vi "default scan size.vi"(0 "data in":T1, 11 "error in":errorcluster) -> (4 "data out":T1, 15 "error out":errorcluster)   [LabVIEW 2013, in "Manipulate IPF.lvlib"]
uses:
  Manipulate IPF.lvlib
  3013/code/Modules/GUI/GUI_5/subPanels/edit/type_def/data.ctl
  3013/code/Modules/Configuration/type_def/Scan Params.ctl
  3013/code/Modules/Configuration/type_def/Profile Resolution.ctl
  3013/code/Modules/Preprocess Data/type_def/direction.ctl
  3013/code/Modules/Inspection/Data/Panel_class/type_def/Config File data.ctl
  3013/code/Modules/Inspection/type_def/Pos and Rot.ctl
  3013/code/Modules/Inspection/Data/PCB_class/type_def/PCB Params.ctl
  3013/code/Modules/Inspection/Data/Panel_class/type_def/BarCode Params.ctl
  3013/code/Modules/Barcode Reader/type_def/id.ctl
  3013/code/Modules/Inspection/Data/Panel_class/type_def/inspection data.ctl
  3013/code/Modules/Inspection/type_def/Range Limits.ctl
  3013/code/Modules/Configuration/Config.lvlib
  3013/code/Modules/Inspection/Inspection.lvlib
  3013/code/Modules/Inspection/Data/PCB_class/PCB.lvclass
  3013/code/Modules/Barcode Reader/Barcode Reader.lvlib
  3013/code/Modules/Inspection/Data/Panel_class/Panel.lvclass
  3013/code/Modules/Preprocess Data/PreProcess.lvlib
  3013/code/Modules/GUI/GUI_5/subPanels/edit/edit.lvlib
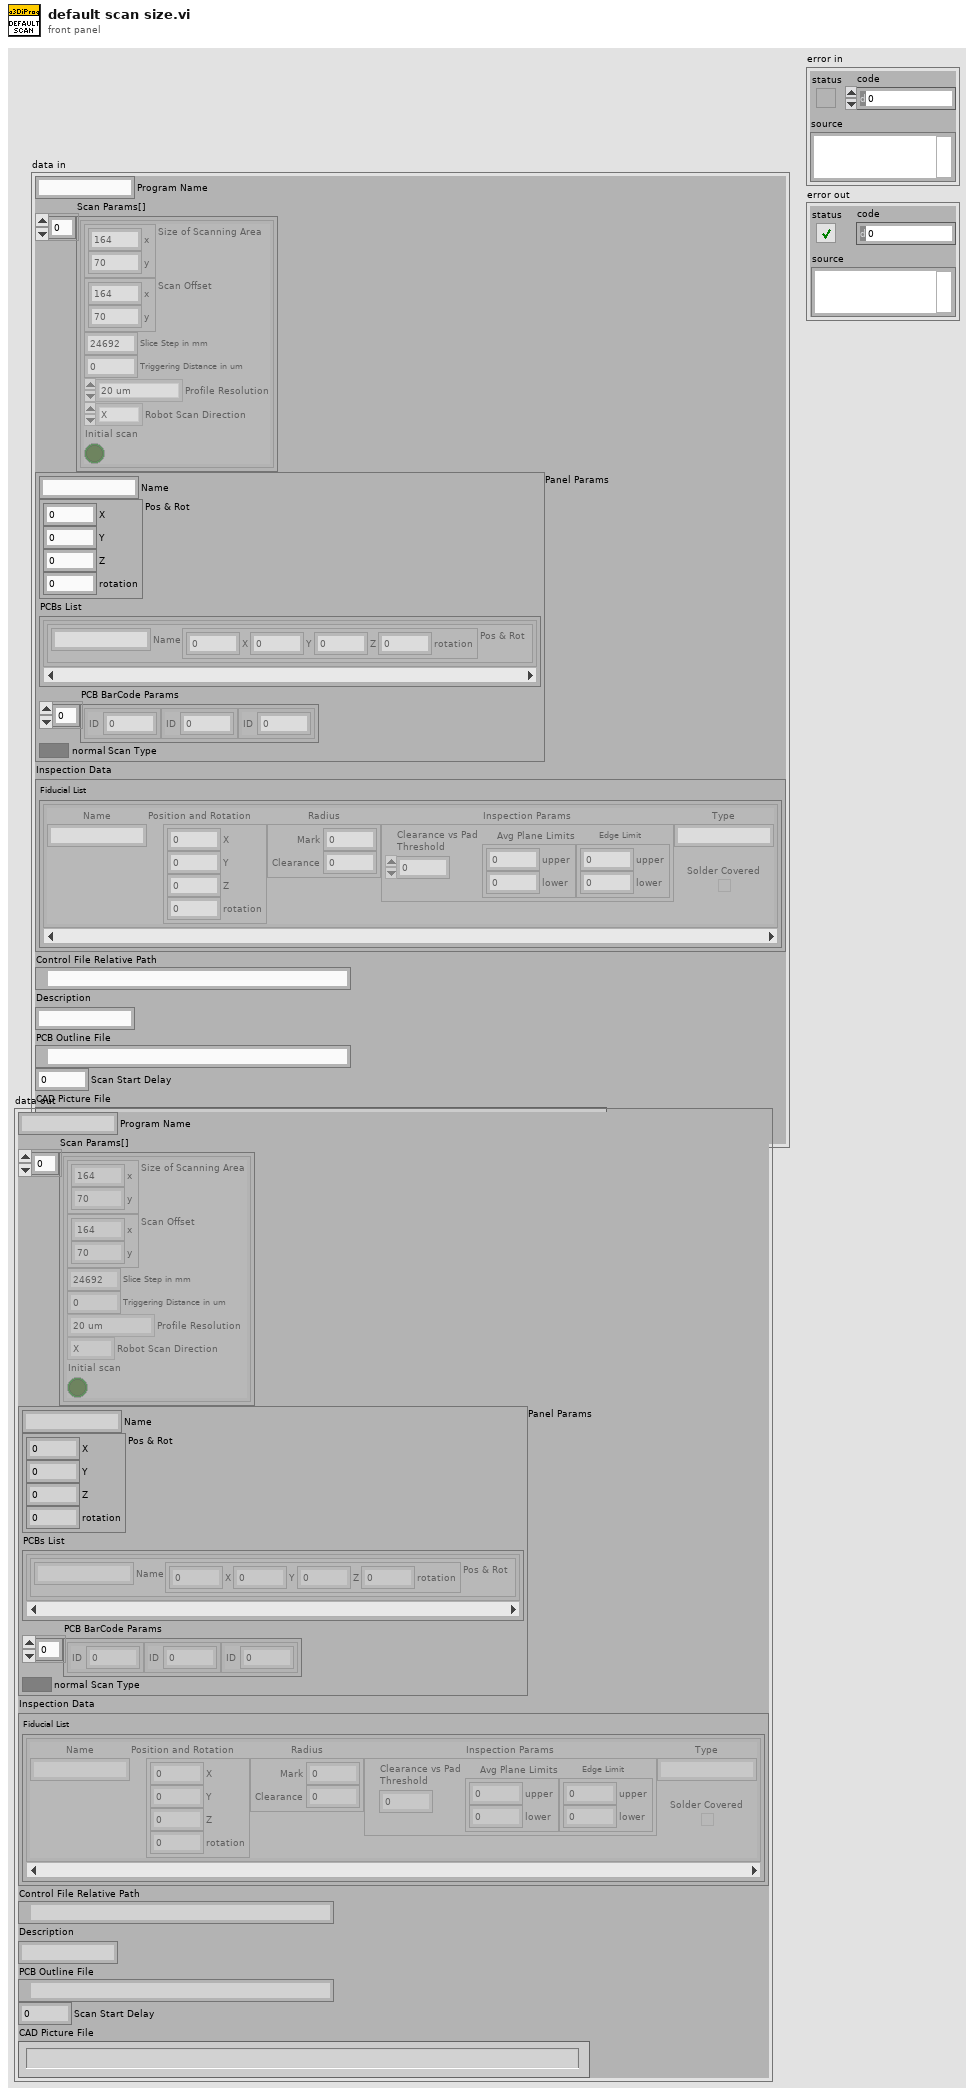
[diagram p1: front panel]
types:
  T1 = typedef "GUI.lvlib/subPanel.lvlib/edit.lvlib/data.ctl" = cluster{"Program Name":string, "Scan Params[]":T2[], "Panel Params":T5, "Inspection Data":T10, "Control File Relative Path":path, "Description":string, "PCB Outline File":path, "Scan Start Delay":dbl, "CAD Picture File":string}
  T2 = typedef "Config.lvlib/Scan Params.ctl" = cluster{"Size of Scanning Area":cluster{"x":dbl, "y":dbl}, "Scan Offset":cluster{"x":dbl, "y":dbl}, "Slice Step in mm":dbl, "Triggering Distance in mm":dbl, "Triggering Distance in um":dbl, "Profile Resolution":T3, "Version":string, "Robot Scan Direction":T4, "Initial scan":bool}
  T3 = typedef "Config.lvlib/Profile Resolution.ctl" = enum8{"20 um", "40 um"}
  T4 = typedef "PreProcess.lvlib/direction.ctl" = enum8{"X", "Y"}
  T5 = typedef "Inspection.lvlib/Panel.lvclass/Config File data.ctl" = cluster{"Name":string, "Pos & Rot":T6, "PCBs List":cluster{"PCB Params":T7}[], "PCB BarCode Params":T8[], "Scan Type":bool}
  T6 = typedef "Inspection.lvlib/Pos and Rot.ctl" = cluster{"X":dbl, "Y":dbl, "Z":dbl, "rotation":dbl}
  T7 = typedef "Inspection.lvlib/PCB.lvclass/PCB Params.ctl" = cluster{"Name":string, "Pos & Rot":T6}
  T8 = typedef "Inspection.lvlib/Panel.lvclass/BarCode Params.ctl" = cluster{"ID":T9}
  T9 = typedef "Barcode Reader.lvlib/id.ctl" = u8
  T10 = typedef "Inspection.lvlib/Panel.lvclass/inspection data.ctl" = cluster{"Fiducial List":cluster{"Name":string, "Position and Rotation":T6, "Radius":cluster{"Mark":dbl, "Clearance":dbl}, "Inspection Params":cluster{"Clearance vs Pad\nThreshold":dbl, "Avg Plane Limits":T11, "Edge Limit":T11}, "Type":string, "Solder Covered":bool}[]}
  T11 = typedef "Inspection.lvlib/Range Limits.ctl" = cluster{"upper":sgl, "lower":sgl}
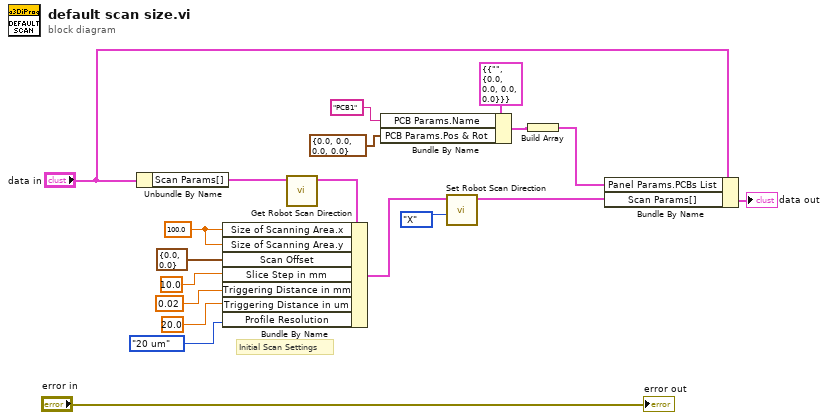
[diagram p0: block diagram]
diagram:
  w11 = 100.0 ("x")
  # "Initial Scan Settings"
  n1 = Unbundle By Name("data in") -> ("Scan Params[]"=w10:T2[])
  n2 = call "Get Robot Scan Direction.vi"("Scan Params[]"=w10) -> ("Scan Params"=w9:T2)  [unwired: 9 in, 1 out]
  n3 = Bundle By Name(cluster=w9, "Size of Scanning Area.x"=w11, "Size of Scanning Area.y"=w11, "Scan Offset"=cluster{"x":dbl, "y":dbl} {"x"=0.0, "y"=0.0} ("Scan Params.Scan Offset"), "Slice Step in mm"=10.0 ("Scan Params.Slice Step in mm"), "Triggering Distance in mm"=0.02 ("Scan Params.Triggering Distance in um"), "Triggering Distance in um"=20.0 ("Scan Params.Triggering Distance in mm"), "Profile Resolution"=Profile_Resolution."20 um" ("Scan Params.Profile Resolution")) -> (w18:T2)
  n4 = Bundle By Name(cluster=cluster{"PCB Params":T7} {"PCB Params"={"Name"="", "Pos & Rot"={"X"=0.0, "Y"=0.0, "Z"=0.0, "rotation"=0.0}}} ("gui"), "PCB Params.Name"="PCB1", "PCB Params.Pos & Rot"=T6 {"X"=0.0, "Y"=0.0, "Z"=0.0, "rotation"=0.0}) -> (w3:cluster{"PCB Params":T7})
  n5 = call "Set Robot Scan Direction.vi"("Scan Direction"=enum32{"X", "Y", "X and Y"}."X" ("Robot Scan Direction"), "Scan Params"=w18) -> ("Scan Params"=w13:T2[])  [unwired: 9 in]
  n6 = Build Array(w3) -> (w5:cluster{"PCB Params":T7}[])
  n7 = Bundle By Name(cluster="data in", "Panel Params.PCBs List"=w5, "Scan Params[]"=w13) -> (→"data out":T1)
  "error out" <- "error in"
